vi "4b - Read global.vi"() -> ()   [LabVIEW 2010]
uses:
  My Globals.vi
panel:
  in  "stop":bool
  out "Chart 2":dbl(graph)
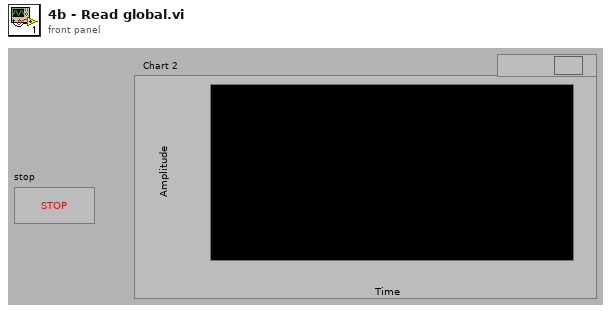
[diagram p1: front panel]
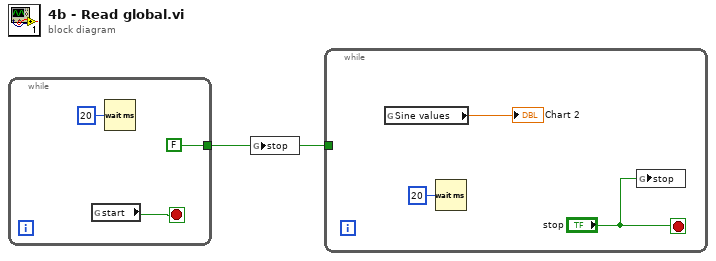
[diagram p0: block diagram]
diagram:
  n1 = while {
    tunnel: [FALSE ("stop")] -> w1
    stop <- w3 stop-if-true
    n2 = global read "My Globals.vi" "start"() -> (w3:bool)
    n3 = Wait (ms)(milliseconds to wait=u32 20) -> ()  [unwired: 1 out]
  }
  n4 = global write "My Globals.vi" "stop"(w1) -> ()
  n5 = while {
    tunnel: w1 -> [_]
    stop <- "stop" stop-if-true
    n6 = global read "My Globals.vi" "Sine values"() -> (→"Chart 2":dbl)
    n7 = Wait (ms)(milliseconds to wait=u32 20) -> ()  [unwired: 1 out]
    n8 = global write "My Globals.vi" "stop"("stop") -> ()
  }
